vi "SetExposure.vi"(8 "error in (no error)":errorcluster, 10 "Setting.Exposure":i32, 11 "DemoCamera in":refnum<class "DemoCamera.lvclass">) -> (0 "error out":errorcluster, 3 "DemoCamera out":refnum<class "DemoCamera.lvclass">)   [LabVIEW 2020, in "DemoCamera.lvlib" / "DemoCamera.lvclass"]
uses:
  DemoCamera.lvclass
  Hardware Abstraction Layer/Component/Camera/Camera/Camera.lvclass
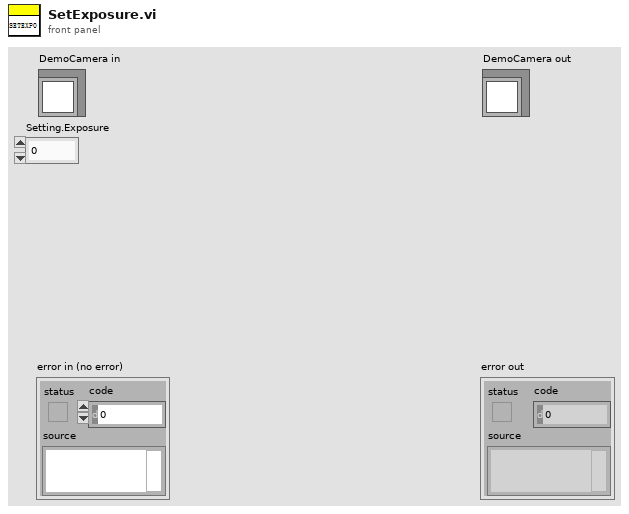
[diagram p1: front panel]
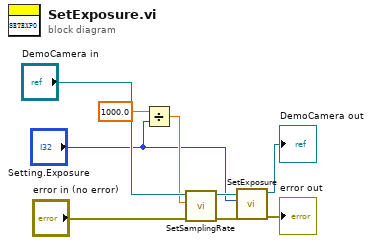
[diagram p0: block diagram]
diagram:
  n1 = Divide(x=1000.0, y="Setting.Exposure") -> (x/y=w3:dbl)
  n2 = call-dynamic "SetSamplingRate.vi"("error in (no error)"="error in (no error)", "SamplingRate(Hz)"=w3, "Device in"="DemoCamera in") -> ("error out"=w6:errorcluster, "Device out"=w4:refnum<class "DemoCamera.lvclass">)  [unwired: 7 in]
  n3 = call-parent "SetExposure.vi"("error in (no error)"=w6, "Setting.Exposure"="Setting.Exposure", "Camera in"=w4) -> ("error out"=→"error out":errorcluster, "Camera out"=→"DemoCamera out":refnum<class "DemoCamera.lvclass">)  [unwired: 7 in]
